vi "Gear.vi"() -> ()   [LabVIEW 2016]
panel:
  in  "Angle Case":i8
  in  "Intake Off":bool
  out "Intake Voltage":dbl
  out "Clamp Voltage":dbl
  in  "Target Angle":dbl
  in  "Gear Loaded":bool
  in  "Current Angle":dbl
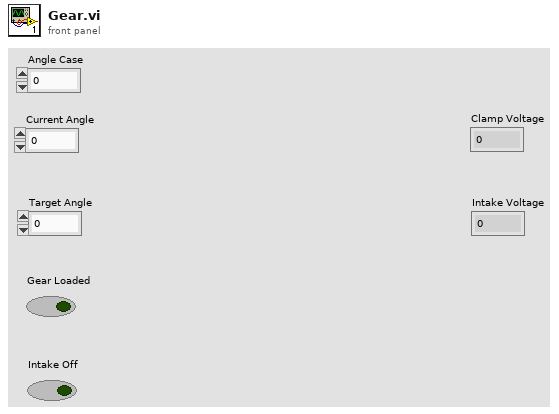
[diagram p1: front panel]
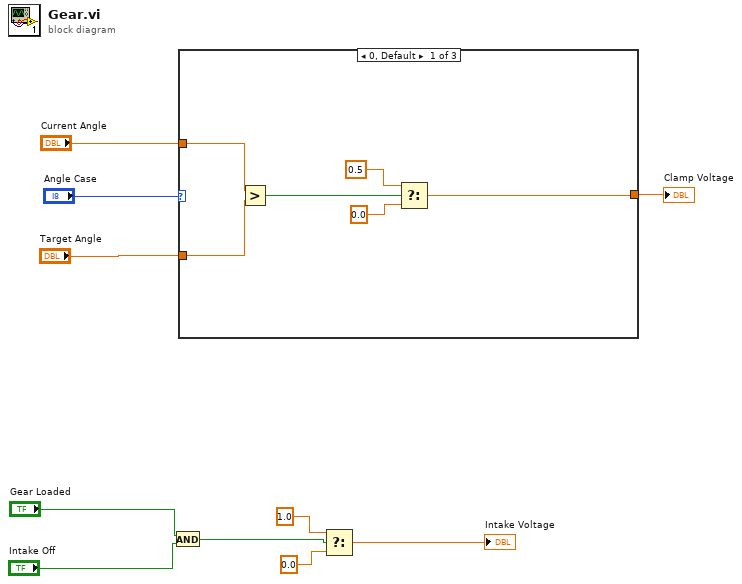
[diagram p0: block diagram]
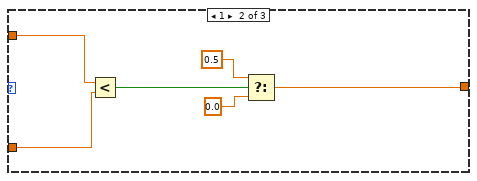
[diagram p2: hidden frame]
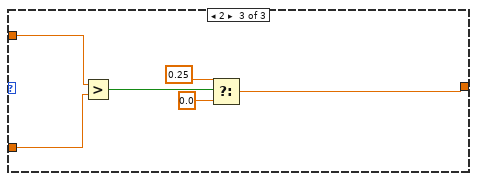
[diagram p3: hidden frame]
diagram:
  n1 = And(x="Gear Loaded", y="Intake Off") -> (x .and. y?=w8:bool)
  n2 = case shown="0, Default" "Angle Case" {
    tunnel: "Current Angle" -> [w16 w22 w28]
    tunnel: "Target Angle" -> [w15 w21 w27]
    tunnel: [w11 w17 w23] -> w1
    frame 0, Default {
      n3 = Greater?(x=w16, y=w15) -> (0:w14:bool)
      n4 = Select(t=0.5, s=w14, f=0.0) -> (s? t:f=w11:dbl)
    }
    frame 1 {
      n5 = Less?(x=w22, y=w21) -> (x < y?=w20:bool)
      n6 = Select(t=0.5, s=w20, f=0.0) -> (s? t:f=w17:dbl)
    }
    frame 2 {
      n7 = Greater?(x=w28, y=w27) -> (0:w26:bool)
      n8 = Select(t=0.25, s=w26, f=0.0) -> (s? t:f=w23:dbl)
    }
  }
  "Clamp Voltage" <- w1
  n9 = Select(t=1.0, s=w8, f=0.0) -> (s? t:f=→"Intake Voltage":dbl)
